vi "Reset Board.vi"(8 "error in (no error)":errorcluster, 11 "CS++GoBangServer in":refnum<class "CS++GoBangServer.lvclass">) -> (0 "error out":errorcluster, 3 "CS++GoBangServer out":refnum<class "CS++GoBangServer.lvclass">)   [LabVIEW 2014, in "GoBang.lvlib" / "CS++GoBangServer.lvclass"]
uses:
  CS++GoBangServer.lvclass
  typdefs/BoardField.ctl
  GoBang.lvlib
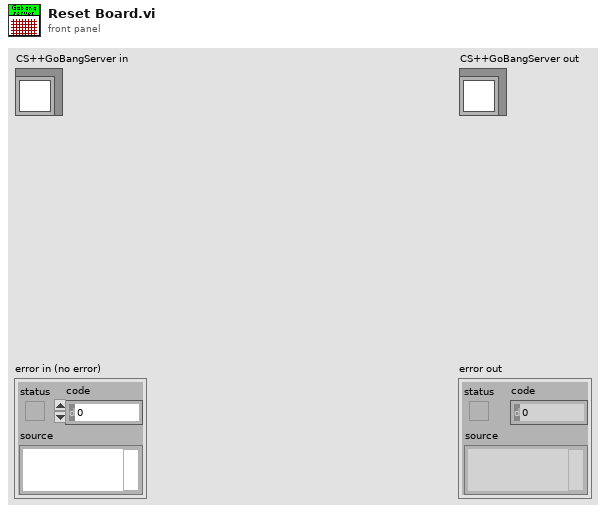
[diagram p1: front panel]
types:
  T1 = typedef "GoBang.lvlib/BoardField.ctl" = u8
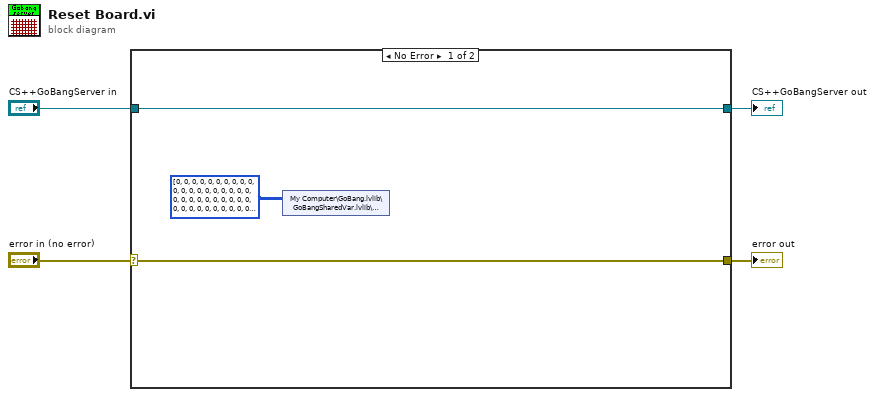
[diagram p0: block diagram]
diagram:
  n1 = case shown="No Error" "error in (no error)" {
    selector: "error in (no error)" -> [w6 w9]
    tunnel: [w6 w9] -> w3
    tunnel: [w7 w8] -> w1
    tunnel: "CS++GoBangServer in" -> [w7 w8]
    frame No Error {
      n2 = shared-variable "My Computer\\GoBang.lvlib\\GoBangSharedVar.lvlib\\GameBoard"(T1[][] [[0, 0, 0, 0, 0, 0, 0, 0, 0, 0], [0, 0, 0, 0, 0, 0, 0, 0, 0, 0], [0, 0, 0, 0, 0, 0, 0, 0, 0, 0], [0, 0, 0, 0, 0, 0, 0, 0, 0, 0], [0, 0, 0, 0, 0, 0, 0, 0, 0, 0], [0, 0, 0, 0, 0, 0, 0, 0, 0, 0], [0, 0, 0, 0, 0, 0, 0, 0, 0, 0], [0, 0, 0, 0, 0, 0, 0, 0, 0, 0], [0, 0, 0, 0, 0, 0, 0, 0, 0, 0], [0, 0, 0, 0, 0, 0, 0, 0, 0, 0]] ("GameBoard")) -> ()  [unwired: 1 in, 1 out]
    }
    frame Error {
    }
  }
  "error out" <- w3
  "CS++GoBangServer out" <- w1
